vi "Reset_All_Relay.vi"(8 "error in (no error)":errorcluster caption="entrée d'erreur (pas d'erreur)", 11 "Class Relay_Board 16_Relay_R4D3D16 en entrée":refnum<class "Class Relay_Board 8_Relay_N4D8B08.lvclass">) -> (0 "error out":errorcluster caption="sortie d'erreur", 3 "Class Relay_Board 16_Relay_R4D3D16 en sortie":refnum<class "Class Relay_Board 8_Relay_N4D8B08.lvclass">)   [LabVIEW 2020, in "Library Instrument & Equipement.lvlib" / "Library Relay_Board.lvlib" / "Class Relay_Board 8_Relay_N4D8B08.lvclass"]
uses:
  Class Relay_Board 8_Relay_N4D8B08.lvclass
  Class Relay_Board 8_Relay_N4D8B08.lvclass/Class Relay_Board 8_Relay_N4D8B08.ctl
  Commun VI/TypeDef/Liste Error.ctl
  Modbus/Modbus.lvclass
  Commun VI/Library Commun.lvlib
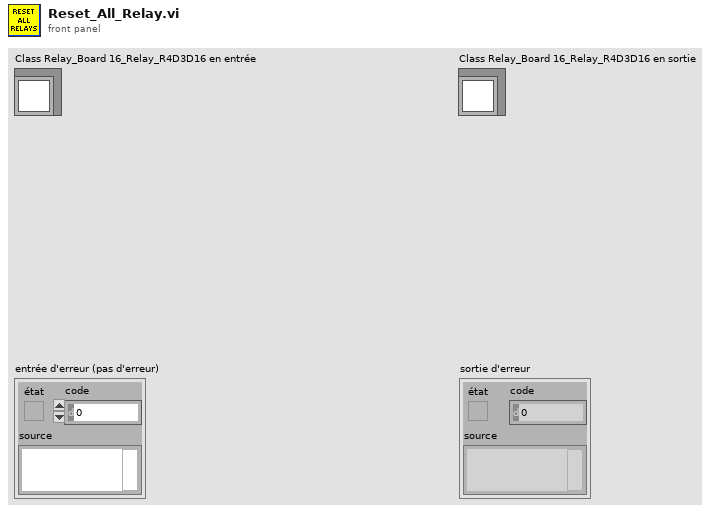
[diagram p1: front panel]
types:
  T1 = typedef "Library Commun.lvlib/Liste Error.ctl" = enum16{"Firebase Driver - Get Document", "Firebase Driver - Get Document With Where", "Firebase Driver - Delete Document", "Firebase Driver - Set Document", "Firebase Driver - Update Document", "Firebase Altyor - Search Document Bench", "Firebase Altyor - Class Not in Firebase", "Spectrum_Analyser - Timeout", "Relay Board - Qty Relay", "DIO - Pb Funtion", "Power_Supply - Peripherical not find", "Mutimeter - Peripherical not find", "Instrument - Function Not Used", "Instrument - Instrument name not specified", "Instrument - Allready Initialised", "Instrument - TimeOut", "Instrument - the instrument must be Initialise before", "Instrument - Frame Not received", "Instrument - Frame Nok", "Test - Initialise the File_for_Save", "Test - Timeout", "Test - Cmd Error", "FGV - Variable ", "BDD FireBase - Define Class", "SN - Class Not Define"}
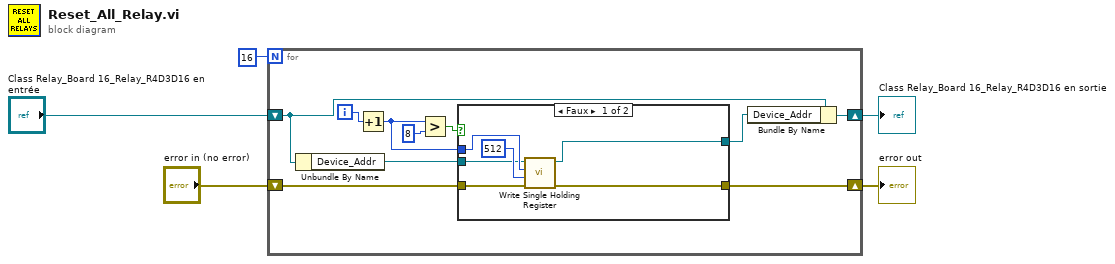
[diagram p0: block diagram]
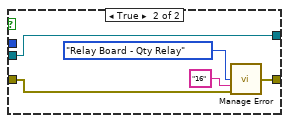
[diagram p2: hidden frame]
diagram:
  n1 = for {
    N: 16 -> [_]
    shift-right: [w14] -> w1
    shift-left: "error in (no error)" -> [w15]
    shift-right: [w9] -> w4
    shift-left: "Class Relay_Board 16_Relay_R4D3D16 en entrée" -> [w11]
    i -> [w7]
    n2 = Unbundle By Name(w11) -> ("Device_Addr"=w8:refnum<class "Modbus.lvclass">)
    n3 = Increment(x=w7) -> (x+1=w6:i32)
    n4 = Greater?(x=w6, y=u8 8) -> (0:w12:bool)
    n5 = case shown="Faux" w12 {
      tunnel: w15 -> [w21 w22]
      tunnel: w6 -> [w20 _]
      tunnel: [w16 w24] -> w14
      tunnel: [w18 w23] -> w10
      tunnel: w8 -> [w17 w23]
      frame False {
        n6 = call "Write Single Holding Register.vi"("error in (no error)"=w21, "value"=u16 512, "address"=w20, "MODBUS in"=w17) -> ("error out"=w16:errorcluster, "MODBUS Out"=w18:refnum<class "Modbus.lvclass">)  [unwired: 6 in]
      }
      frame True {
        n7 = call "Manage Error.vi"("Code Erreur"=Liste_Error."Relay Board - Qty Relay", "Text"="16", "error in (no error)"=w22) -> ("error out"=w24:errorcluster)  [unwired: 12 in]
      }
    }
    n8 = Bundle By Name(cluster=w11, "Device_Addr"=w10) -> (w9:refnum<class "Class Relay_Board 8_Relay_N4D8B08.lvclass">)
  }
  "error out" <- w1
  "Class Relay_Board 16_Relay_R4D3D16 en sortie" <- w4
